vi "Unregister Q.vi"(8 "error in (no error)":errorcluster, 10 "Q Number":i32, 11 "VolatusAPI in":refnum<class "VolatusAPI.lvclass">) -> (0 "error out":errorcluster, 3 "VolatusAPI out":refnum<class "VolatusAPI.lvclass">)   [LabVIEW 2020, in "Volatus.lvlib" / "VolatusAPI.lvclass"]
uses:
  VolatusAPI.lvclass
  VolatusAPI.lvclass/VolatusAPI.ctl
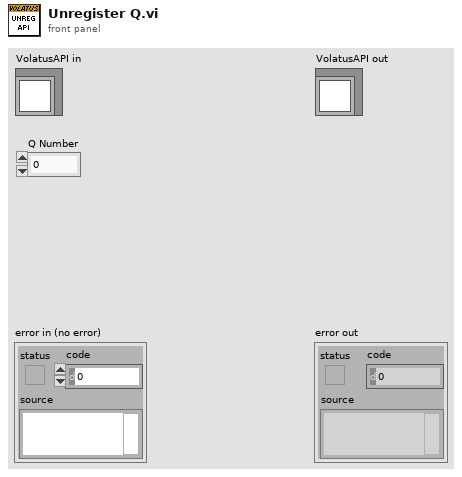
[diagram p1: front panel]
types:
  T1 = typedef "Volatus.lvlib/VolatusAPI.lvclass/MsgQs Ref.ctl" = cluster{"Keys":map{string, T2}, "MsgQs":map{i32, T3}, "Next Number":i32}
  T2 = typedef "Volatus.lvlib/VolatusAPI.lvclass/Q Info.ctl" = cluster{"Number":i32, "Notifiers":refnum<notifier>[]}
  T3 = typedef "Volatus.lvlib/VolatusAPI.lvclass/Registered Q.ctl" = cluster{"Q":refnum<class "MessageQ.lvclass">, "Keys":string[]}
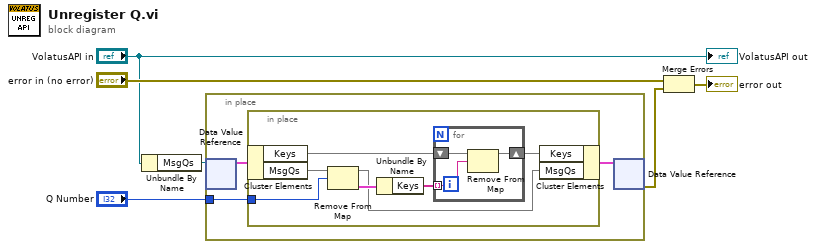
[diagram p0: block diagram]
diagram:
  n1 = Unbundle By Name("VolatusAPI in") -> ("MsgQs"=w5:refnum<data-value>)
  n2 = in-place {
    in-place-border: "Q Number" -> [w7]
    n3 = in-place-dvr #1(w5) -> (w9:T1)  [unwired: 1 out]
    n4 = in-place {
      in-place-border: w7 -> [w15]
      n5 = in-place-cluster #2(w9) -> ("Keys"=w13:map{string, T2}, "MsgQs"=w16:map{i32, T3})
      n6 = Remove From Map(10:w15, 11:w16) -> (1:w14:T3, 3:w10:map{i32, T3})  [unwired: 1 out]
      n7 = Unbundle By Name(w14) -> ("Keys"=w12:string[])
      n8 = for {
        shift-right: [w18] -> w11
        shift-left: w13 -> [w19]
        tunnel: w12 -> [w17] mode=indexing
        n9 = Remove From Map(10:w17, 11:w19) -> (3:w18:map{string, T2})  [unwired: 2 out]
      }
      n10 = in-place-cluster #2("Keys"=w11, "MsgQs"=w10) -> (w8:T1)
    }
    n11 = in-place-dvr #1(w8) -> (w1:errorcluster)  [unwired: 1 out]
  }
  n12 = Merge Errors("error in (no error)", w1) -> (→"error out":errorcluster)
  "VolatusAPI out" <- "VolatusAPI in"
